vi "Close.vi"(11 "ADALM2000 Handler":u32 caption="Instrument Handle Out") -> ()   [LabVIEW 2015]
uses:
  libm2k_lv.dll
panel:
  in  "error in (no error)":errorcluster
  out "Error Out":errorcluster
  out "?":dbl format="%#_13g"
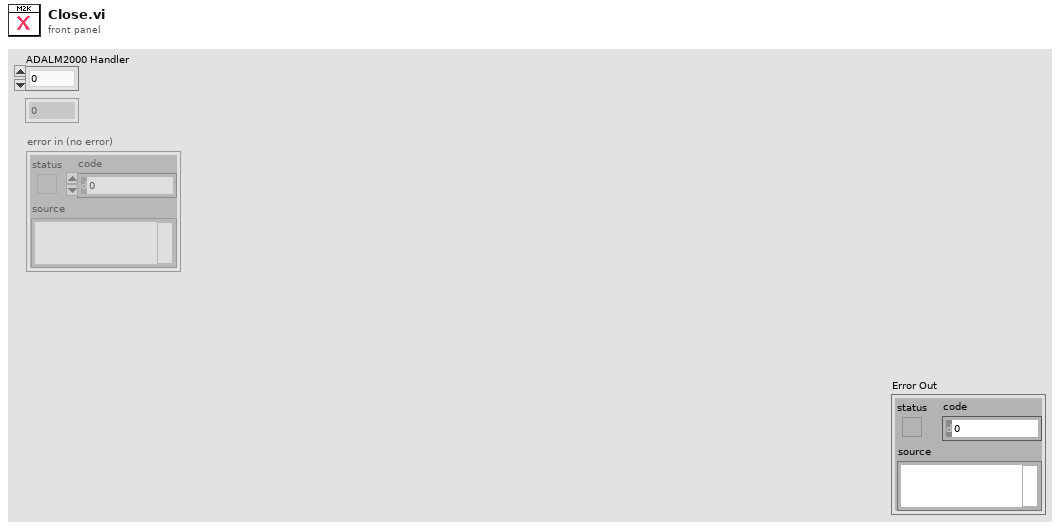
[diagram p1: front panel]
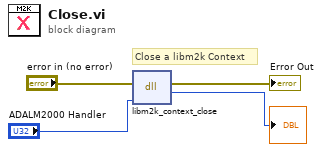
[diagram p0: block diagram]
diagram:
  # "Close a libm2k Context"
  n1 = dll-call lib="libm2k_lv.dll" fn="libm2k_context_close"(error in="error in (no error)", "arg1"="ADALM2000 Handler") -> (error out=→"Error Out":errorcluster, "return type"=→"?":i64)  [unwired: 3 in, 1 out]
